vi "getAIwfm.vi"(8 "error in (no error)":errorcluster, 11 "Instrument.LockinAPI in":refnum<class "Instrument.LockinAPI.lvclass">) -> (0 "error out":errorcluster, 2 "AI Waveform":waveform(dbl)[](array[waveform]), 3 "Instrument.LockinAPI out":refnum<class "Instrument.LockinAPI.lvclass">)   [LabVIEW 2019, in "Instrument.LockinAPI.lvclass"]
doc: "API to get the AI waveforms.\n\nIf address=\"\", this API reads from localhost\nIf address is remote lockin, you need to add this computer to allowed whitelist on the lockin computer you are trying to access."
uses:
  Instrument.LockinAPI.lvclass
  C:/Users/patrick/Documents/GitHub/Instrument-Framework/lvsrc/Instrument/Instrument.lvclass
  Typedefs/API/LockinAPI.Commands--Enum.ctl
  47302476-cf8c-41d6-bca0-f4867c98124e.vi
  47302476-cf8c-41d6-bca0-f4867c98124e.vi/d50d826d-55e5-4a85-a0b1-7a9f3e058d7e.vi
  47302476-cf8c-41d6-bca0-f4867c98124e.vi/d50d826d-55e5-4a85-a0b1-7a9f3e058d7e.vi/6a9065c5-a83d-4d1b-8b71-0acf588a60b9.vi
  47302476-cf8c-41d6-bca0-f4867c98124e.vi/d50d826d-55e5-4a85-a0b1-7a9f3e058d7e.vi/0ae1e62a-96e1-4e0f-83f1-a12d225e976f.vi
  47302476-cf8c-41d6-bca0-f4867c98124e.vi/d50d826d-55e5-4a85-a0b1-7a9f3e058d7e.vi/422ad838-5cfd-4770-b268-e735c1942843.vi
  <vilib>/JDP Science/JSONtext/Make JSON Array.vi
  47302476-cf8c-41d6-bca0-f4867c98124e.vi/d50d826d-55e5-4a85-a0b1-7a9f3e058d7e.vi/0ae1e62a-96e1-4e0f-83f1-a12d225e976f.vi/d2e2794b-fcb6-4cf8-bcf6-983bc4ba0092.vi
  47302476-cf8c-41d6-bca0-f4867c98124e.vi/d50d826d-55e5-4a85-a0b1-7a9f3e058d7e.vi/422ad838-5cfd-4770-b268-e735c1942843.vi/30eaffc9-1ec5-4bf4-9010-3724b7ccfc0c.vi
  47302476-cf8c-41d6-bca0-f4867c98124e.vi/d50d826d-55e5-4a85-a0b1-7a9f3e058d7e.vi/422ad838-5cfd-4770-b268-e735c1942843.vi/e3d86699-460e-4ceb-921f-23802032ce75.vi
  Instrument/API/Enum to String.vi
  Instrument/Private/Get RC Connection Status.vi
  <vilib>/JDP Science/JSONtext/Variant to JSON Text.vi
  <vilib>/JDP Science/JSONtext/support/Format JSON Array Text.vi
  Instrument/API/Send and Receive.vi
  <vilib>/JDP Science/JSONtext/JSON text to Variant.vi
  <vilib>/Utility/Data Type/Get Type Information.vi
  <vilib>/JDP Science/JSONtext/LVClass Serializer/JSONtext LVClass Serializer.lvclass
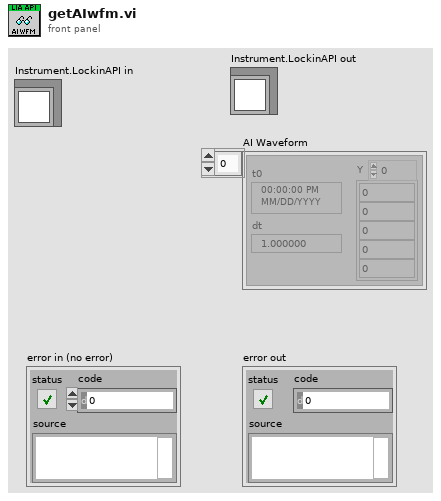
[diagram p1: front panel]
types:
  T1 = typedef "Instrument.LockinAPI.lvclass/LockinAPI.Commands--Enum.ctl" = enum16{"setAI", "setAO", "setAO_Amplitude", "setAO_DC", "setAO_Frequency", "setAO_Phase", "setAO_Function", "setAO_I+", "setREF", "setREF_Frequency", "setREF_Phase", "setREF_TC", "setREF_Roll-Off", "setDAQ", "setSampling", "setOffset", "setState", "getState", "getAO", "getAI", "getResults", "getSampling", "getAOconfig", "getREFconfig", "setInputGain", "setOutputGain", "getInputGain", "getOutputGain", "setSamplingMode", "getSamplingMode", "setSweep", "setSweepTime", "setSweepTable", "getStatus", "getSweepResults", "getSweepWaveforms", "startSweep", "stopSweep", "setAUX", "getAUX"}
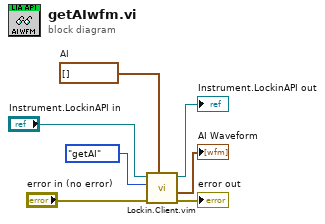
[diagram p0: block diagram]
diagram:
  w7 = waveform(dbl)[] []  # AI
  n1 = call "Lockin.Client.vim"("Data Out type"=w7, "error in (no error)"="error in (no error)", "Command"=LockinAPI.Commands--Enum."getAI", "Instrument.LockinAPI in"="Instrument.LockinAPI in") -> ("error out"=→"error out":errorcluster, "Data out"=→"AI Waveform":waveform(dbl)[], "Instrument.LockinAPI out"=→"Instrument.LockinAPI out":refnum<class "Instrument.LockinAPI.lvclass">)  [unwired: 5 in]
